vi "ConvLongTemps.vi"(0 "Input Units":i8(ring) items=["mm", "ps"], 5 "Units Input":dbl caption="Input (Units)", 9 "Output Units":i8(ring) items=["mm", "ps"], 11 "error in (no error)":errorcluster caption="entrée d'erreur (pas d'erreur)") -> (4 "Units Output":dbl caption="Output (Units)", 6 "Units mm":dbl caption="mm out", 8 "Units ps":dbl caption="ps out", 15 "error out":errorcluster caption="sortie d'erreur")   [LabVIEW 2010]
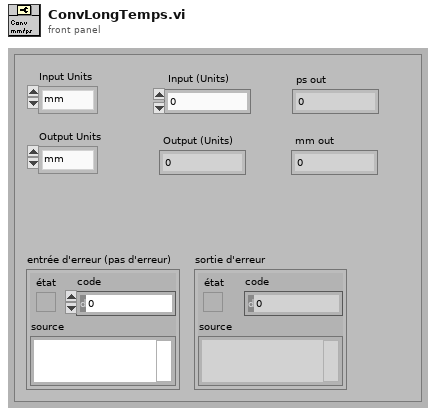
[diagram p1: front panel]
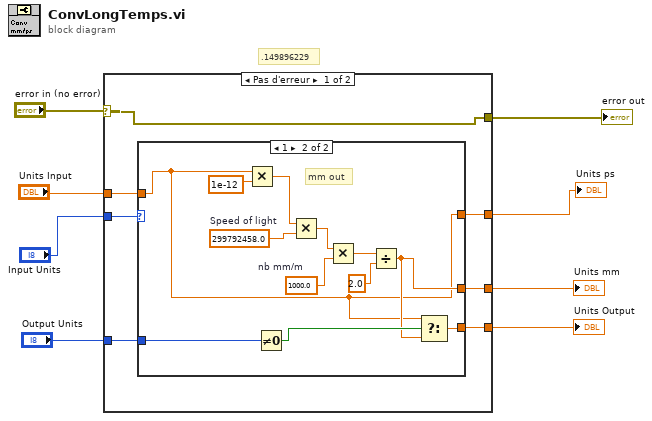
[diagram p0: block diagram]
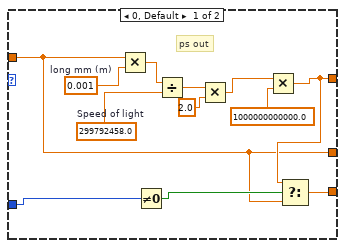
[diagram p2: hidden frame]
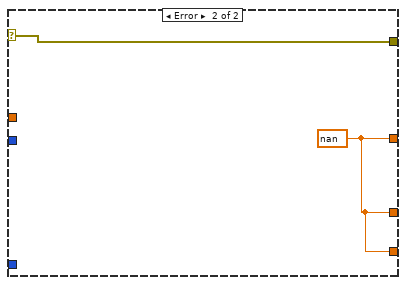
[diagram p3: hidden frame]
diagram:
  # ".149896229"
  n1 = case shown="Pas d'erreur" "error in (no error)" {
    selector: "error in (no error)" -> [w15 w41]
    tunnel: [w15 w41] -> w7
    tunnel: "Input Units" -> [w14 _]
    tunnel: "Units Input" -> [w13 _]
    tunnel: [w12 w40] -> w4
    tunnel: [w11 w40] -> w3
    tunnel: "Output Units" -> [w10 _]
    tunnel: [w9 w40] -> w1
    frame No Error {
      n2 = case shown="1" w14 {
        tunnel: w13 -> [w16 w28]
        tunnel: [w17 w28] -> w12
        tunnel: [w16 w29] -> w11
        tunnel: w10 -> [w19 w31]
        tunnel: [w20 w32] -> w9
        frame 0, Default {
          w24 = 0.001  # long mm (m)
          w21 = 299792458.0  # Speed of light
          # "ps out"
          n3 = Multiply(x=w16, y=w24) -> (x*y=w25:dbl)
          n4 = Not Equal To 0?(x=w19) -> (x != 0?=w18:bool)
          n5 = Divide(x=w25, y=w21) -> (x/y=w22:dbl)
          n6 = Multiply(x=w22, y=2.0) -> (x*y=w26:dbl)
          n7 = Multiply(x=w26, y=1000000000000.0) -> (x*y=w17:dbl)
          n8 = Select(t=w17, s=w18, f=w16) -> (s? t:f=w20:dbl)
        }
        frame 1 {
          w37 = 1000.0  # nb mm/m
          w36 = 299792458.0  # Speed of light
          # "mm out"
          n9 = Multiply(x=w28, y=1e-12) -> (x*y=w39:dbl)
          n10 = Not Equal To 0?(x=w31) -> (x != 0?=w30:bool)
          n11 = Multiply(x=w39, y=w36) -> (x*y=w35:dbl)
          n12 = Multiply(x=w35, y=w37) -> (x*y=w33:dbl)
          n13 = Divide(x=w33, y=2.0) -> (x/y=w29:dbl)
          n14 = Select(t=w28, s=w30, f=w29) -> (s? t:f=w32:dbl)
        }
      }
    }
    frame Error {
      w40 = nan
    }
  }
  "error out" <- w7
  "Units ps" <- w4
  "Units mm" <- w3
  "Units Output" <- w1
